vi "Scan Engine Initialization VI.vi"(8 "error in (no error)":errorcluster, 10 "Custom XML":string, 11 "Device Item Ref in":T1 format="%.0x") -> (0 "error out":errorcluster, 3 "Device Item Ref out":T1 format="%.0x")   [LabVIEW 2024, in "SEECD System Explorer.lvlib"]
uses:
  SEECD System Explorer.lvlib
  <vilib>/NI VeriStand/Custom Device API/Custom Device Item Ref.ctl
  <vilib>/NI VeriStand/Custom Device API/Custom Device Channel.ctl
  <vilib>/NI VeriStand/Custom Device API/Custom Device Channel Type.ctl
  Shared/Globals/Property Strings.vi
  <vilib>/NI VeriStand/Custom Device API/Set Item Property (U16).vi
  <vilib>/NI VeriStand/Custom Device API/Custom Device API.lvlib
  Shared/SEECD Shared.lvlib
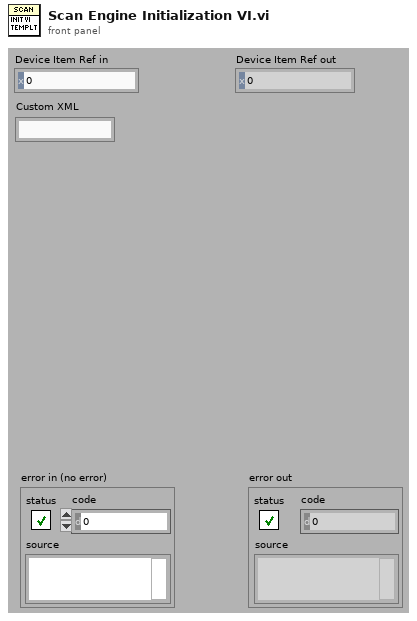
[diagram p1: front panel]
types:
  T1 = typedef "Custom Device API.lvlib/Custom Device Item Ref.ctl" = u64
  T2 = typedef "Custom Device API.lvlib/Custom Device Channel.ctl" = cluster{"Type":T3, "Units":string, "Default Value":dbl, "Faultable":bool, "Scalable":bool}
  T3 = typedef "Custom Device API.lvlib/Custom Device Channel Type.ctl" = enum16{"Input", "Output"}
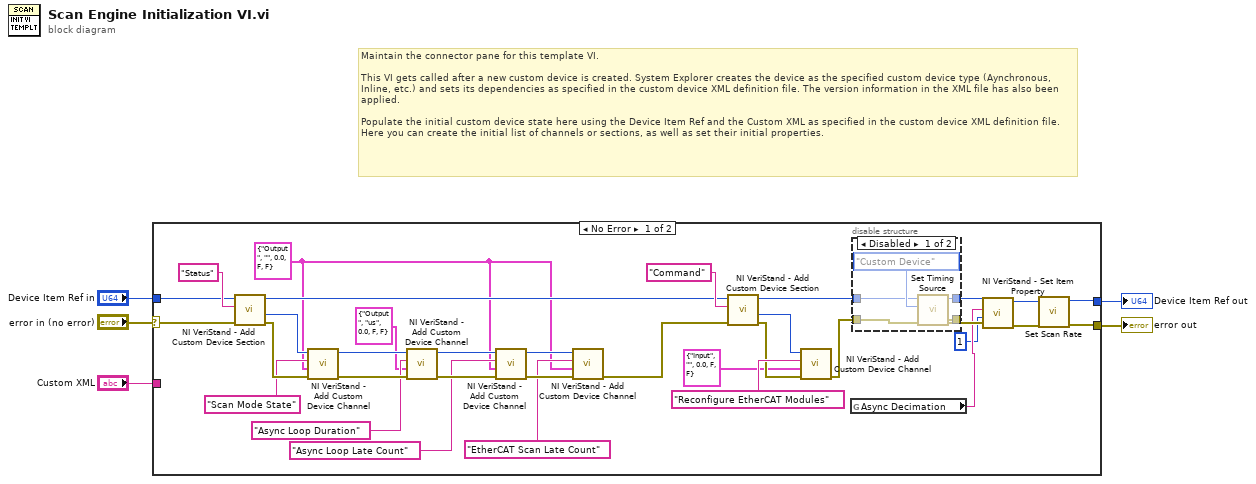
[diagram p0: block diagram]
diagram:
  # "Maintain the connector pane for this template VI.\n\nThis VI gets called after a new custom device is created. System Explorer creates the device as the specified custom device type (Aynchronous, Inline, etc.) and sets its dependencies as specified in the custom device XML definition file. The version information in the XML file has also been applied.\n\nPopulate the initial custom device state here using the Device Item Ref and the Custom XML as specified in the custom device XML definition file. Here you can create the initial list of channels or sections, as well as set their initial properties."
  n1 = case shown="No Error" "error in (no error)" {
    selector: "error in (no error)" -> [w22 w48]
    tunnel: [w8 w48] -> w5
    tunnel: [w7 w47] -> w3
    tunnel: "Device Item Ref in" -> [w23 w47]
    tunnel: "Custom XML" -> [_ _]
    frame No Error {
      w10 = T2 {"Type"=enum."Output", "Units"="", "Default Value"=0.0, "Faultable"=FALSE, "Scalable"=FALSE} ("Channel")
      n2 = call <vilib>:"NI VeriStand - Add Custom Device Section.vi"("error in (no error)"=w22, "Section Name"="Status", "Parent Ref in"=w23) -> ("error out"=w37:errorcluster, "Section Ptr"=w38:T1, "Parent Ref out"=w30:T1)  [unwired: 5 in, 1 out]
      n3 = call <vilib>:"NI VeriStand - Add Custom Device Channel.vi"("error in (no error)"=w37, "Channel"=w10, "Channel Name"="Scan Mode State", "Parent Ref in"=w38) -> ("error out"=w21:errorcluster, "Parent Ref out"=w18:T1)  [unwired: 4 in, 2 out]
      n4 = call <vilib>:"NI VeriStand - Add Custom Device Channel.vi"("error in (no error)"=w21, "Channel"=T2 {"Type"=enum."Output", "Units"="us", "Default Value"=0.0, "Faultable"=FALSE, "Scalable"=FALSE}, "Channel Name"="Async Loop Duration", "Parent Ref in"=w18) -> ("error out"=w20:errorcluster, "Parent Ref out"=w19:T1)  [unwired: 4 in, 2 out]
      n5 = call <vilib>:"NI VeriStand - Add Custom Device Channel.vi"("error in (no error)"=w20, "Channel"=w10, "Channel Name"="Async Loop Late Count", "Parent Ref in"=w19) -> ("error out"=w14:errorcluster, "Parent Ref out"=w15:T1)  [unwired: 4 in, 2 out]
      n6 = call <vilib>:"NI VeriStand - Add Custom Device Channel.vi"("error in (no error)"=w14, "Channel"=w10, "Channel Name"="EtherCAT Scan Late Count", "Parent Ref in"=w15) -> ("error out"=w12:errorcluster)  [unwired: 4 in, 3 out]
      n7 = call <vilib>:"NI VeriStand - Add Custom Device Section.vi"("error in (no error)"=w12, "Section Name"="Command", "Parent Ref in"=w30) -> ("error out"=w34:errorcluster, "Section Ptr"=w33:T1, "Parent Ref out"=w29:T1)  [unwired: 5 in, 1 out]
      n8 = call <vilib>:"NI VeriStand - Add Custom Device Channel.vi"("error in (no error)"=w34, "Channel"=T2 {"Type"=enum."Input", "Units"="", "Default Value"=0.0, "Faultable"=FALSE, "Scalable"=FALSE}, "Channel Name"="Reconfigure EtherCAT Modules", "Parent Ref in"=w33) -> ("error out"=w28:errorcluster)  [unwired: 4 in, 3 out]
      n9 = global read "Property Strings.vi" "Async Decimation"() -> (w25:string)
      n10 = disable-structure shown="Disabled" {
        disable-tunnel: w29 -> [w43 w46]
        disable-tunnel: w28 -> [w42 w45]
        disable-tunnel: [w41 w46] -> w27
        disable-tunnel: [w40 w45] -> w26
        frame Disabled {
          n11 = call "Set Timing Source.vi"("error in (no error)"=w42, "Timing Source"=enum16{"Automatic", "Custom Device"}."Custom Device", "Item Ref in"=w43) -> ("error out"=w40:errorcluster, "Item Ref out"=w41:T1)  [unwired: 7 in]
        }
        frame Enabled {
        }
      }
      n12 = call-poly <vilib>:"NI VeriStand - Set Item Property.vi"("error in (no error)"=w26, "Value"=u16 1, "Property Name"=w25, "Item Ref in"=w27) -> ("error out"=w9:errorcluster, "Item Ref out"=w6:T1)  [unwired: 5 in, 1 out]
      n13 = call "Set Scan Rate.vi"("error in (no error)"=w9, "Device Item Ref in"=w6) -> ("error out"=w8:errorcluster, "Device Item Ref out"=w7:T1)  [unwired: 7 in, 1 out]
    }
    frame Error {
    }
  }
  "error out" <- w5
  "Device Item Ref out" <- w3
